vi "VI Tree.vi"   [LabVIEW 2012, in "MicroStrain 3DM-GXx.lvlib"]
doc: "This is the instrument driver for the MicroStrain 3DM-GX2 and 3DM-GX3 inertial measurment units. The VI Tree displays all the user-callable VIs of the instrument driver in an organized table."
uses:
  <instrlib>/MicroStrain 3DM-GXx/MicroStrain 3DM-GXx.lvlib
  <instrlib>/MicroStrain 3DM-GXx/Public/Data/Parse Message VIs/Parse (Euler Angles).vi
  <instrlib>/MicroStrain 3DM-GXx/Public/Data/Read Single Measurement/Read (Euler Angles).vi
panel:
  # "(c) 2009 - 2011 National Instruments.  ALL RIGHTS RESERVED."
  # "SEE DIAGRAM\nFOR VI TREE."
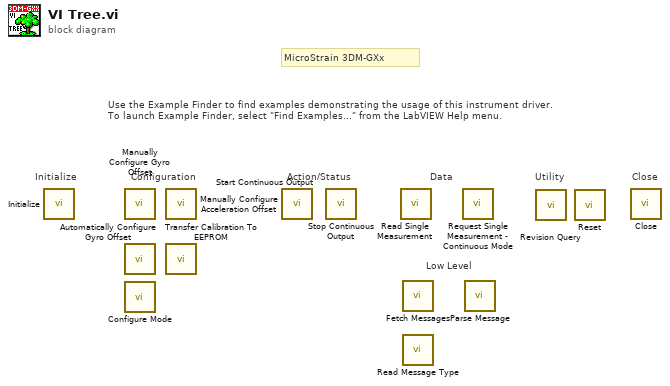
[diagram p0: block diagram]
diagram:
  # "Low Level"
  # "MicroStrain 3DM-GXx"
  # "Use the Example Finder to find examples demonstrating the usage of this instrument driver.\nTo launch Example Finder, select \"Find Examples...\" from the LabVIEW Help menu."
  # "Configuration"
  # "Utility"
  # "Data"
  # "Action/Status"
  # "Close"
  # "Initialize"
  n1 = call <instrlib>:"Initialize.vi"() -> ()  [unwired: 10 in, 2 out]
  n2 = call <instrlib>:"Manually Configure Gyro Offset.vi"() -> ()  [unwired: 14 in, 2 out]
  n3 = call <instrlib>:"Automatically Configure Gyro Offset.vi"() -> ()  [unwired: 10 in, 2 out]
  n4 = call <instrlib>:"Configure Mode.vi"() -> ()  [unwired: 10 in, 2 out]
  n5 = call <instrlib>:"Manually Configure Acceleration Offset.vi"() -> ()  [unwired: 14 in, 2 out]
  n6 = call <instrlib>:"Transfer Calibration To EEPROM.vi"() -> ()  [unwired: 10 in, 2 out]
  n7 = call <instrlib>:"Start Continuous Output.vi"() -> ()  [unwired: 14 in, 2 out]
  n8 = call <instrlib>:"Stop Continuous Output.vi"() -> ()  [unwired: 10 in, 2 out]
  n9 = call-poly <instrlib>:"Read Single Measurement.vi"() -> ()  [unwired: 9 in, 7 out]
  n10 = call <instrlib>:"Fetch Messages.vi"() -> ()  [unwired: 8 in, 4 out]
  n11 = call <instrlib>:"Read Message Type.vi"() -> ()  [unwired: 11 in, 1 out]
  n12 = call <instrlib>:"Request Single Measurement - Continuous Mode.vi"() -> ()  [unwired: 14 in, 2 out]
  n13 = call-poly <instrlib>:"Parse Message.vi"() -> ()  [unwired: 12 in, 4 out]
  n14 = call <instrlib>:"Revision Query.vi"() -> ()  [unwired: 8 in, 4 out]
  n15 = call <instrlib>:"Reset.vi"() -> ()  [unwired: 10 in, 2 out]
  n16 = call <instrlib>:"Close.vi"() -> ()  [unwired: 11 in, 1 out]
